vi "Set Configuration.vi"(8 "error in (no error)":errorcluster, 11 "EST Digital Event in":refnum<class "Digital Event.lvclass">) -> (0 "error out":errorcluster, 3 "EST Digital Event out":refnum<class "Digital Event.lvclass">)   [LabVIEW 2015, in "Digital Event.lvclass"]
uses:
  Digital Event.lvclass
  IO Class/Type.ctl
  EST Input/EST Input.lvclass
  IO Class/IO Class.lvclass
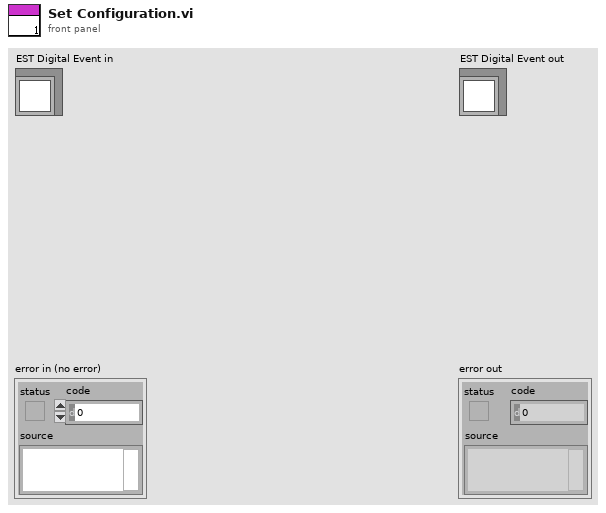
[diagram p1: front panel]
types:
  T1 = typedef "IO Class.lvclass/Type.ctl" = cluster{"Type":string}
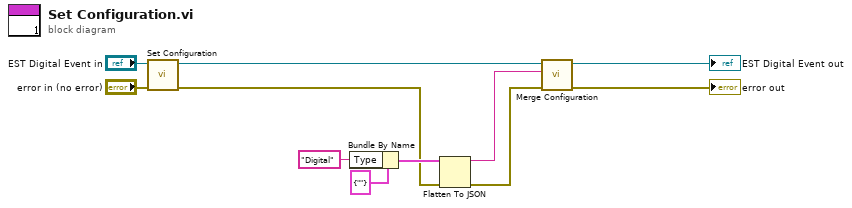
[diagram p0: block diagram]
diagram:
  n1 = call-parent "Set Configuration.vi"("error in (no error)"="error in (no error)", "EST Input in"="EST Digital Event in") -> ("error out"=w4:errorcluster, "EST Input out"=w2:refnum<class "Digital Event.lvclass">)  [unwired: 8 in]
  n2 = Bundle By Name(cluster=T1 {"Type"=""} ("Type"), "Type"="Digital") -> (w8:T1)
  n3 = Flatten To JSON(anything=w8, error in (no error)=w4) -> (JSON string=w7:string, 11:w6:errorcluster)  [unwired: 1 in]
  n4 = call "Merge Configuration.vi"("error in (no error)"=w6, "Additional Configuration"=w7, "IO Class in"=w2) -> ("error out"=→"error out":errorcluster, "IO Class out"=→"EST Digital Event out":refnum<class "Digital Event.lvclass">)  [unwired: 7 in]
